vi "Register with Volatus API.vi"(8 "error in (no error)":errorcluster, 11 "Volatus Core in":refnum<class "Volatus Core.lvclass">) -> (0 "error out":errorcluster, 3 "Volatus Core out":refnum<class "Volatus Core.lvclass">)   [LabVIEW 2020, in "Volatus.lvlib" / "Volatus Core.lvclass"]
uses:
  Volatus Core.lvclass
  Volatus Core.lvclass/Volatus Core.ctl
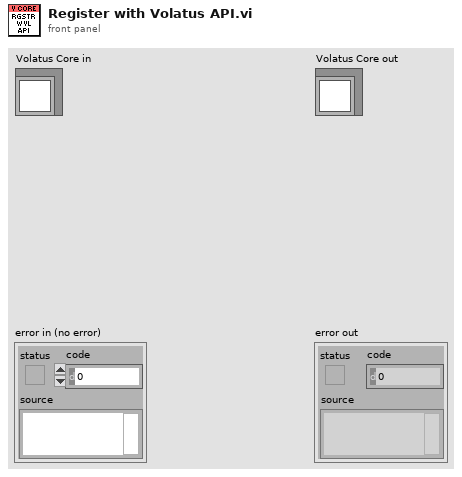
[diagram p1: front panel]
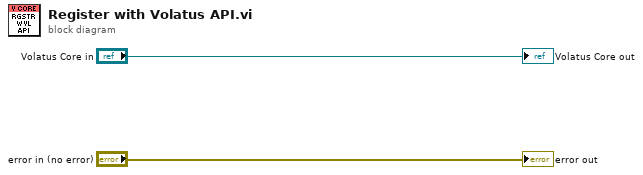
[diagram p0: block diagram]
diagram:
  "error out" <- "error in (no error)"
  "Volatus Core out" <- "Volatus Core in"
